vi "Validate DAQ model.vi"(8 "error in (no error)":errorcluster, 10 "Desired model":string[](array[string]), 11 "DAQ Module ID":i32) -> (0 "error out":errorcluster, 2 "Device found":string, 3 "Is model valid?":bool)   [LabVIEW 2020]
doc: "Validates whether the DAQ connected at the port is a desired DAQ model."
uses:
  NI_DAQ/Libraries/NI DAQ/NI DAQ.lvlib
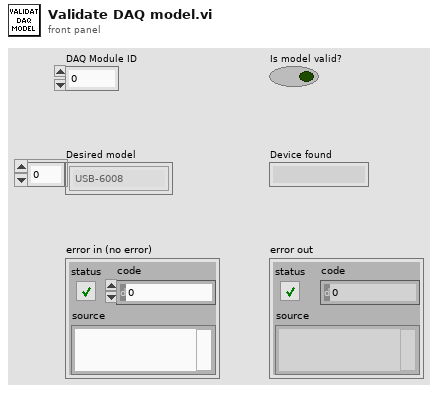
[diagram p1: front panel]
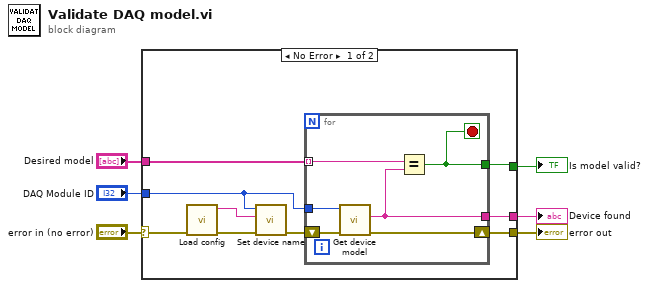
[diagram p0: block diagram]
diagram:
  n1 = case shown="No Error" "error in (no error)" {
    selector: "error in (no error)" -> [w10 w22]
    tunnel: [w7 _] -> w6
    tunnel: "DAQ Module ID" -> [w15 _]
    tunnel: [w14 w22] -> w4
    tunnel: "Desired model" -> [w8 _]
    tunnel: [w9 _] -> w1
    frame No Error {
      n2 = call "Load config.vi"("error in (no error)"=w10) -> ("error out"=w11:errorcluster, "DAQ Port"=w12:tag)  [unwired: 9 in]
      n3 = call "Set device name.vi"("error in"=w11, "Device name"=w12, "Module ID"=w15) -> ("error out"=w13:errorcluster)  [unwired: 8 in]
      n4 = for {
        tunnel: w15 -> [w21]
        tunnel: [w17] -> w9
        shift-right: [w20] -> w14
        shift-left: w13 -> [w19]
        tunnel: w8 -> [w18] mode=indexing
        tunnel: [w16] -> w7
        stop <- w16 stop-if-true
        n5 = call "Get device model.vi"("error in"=w19, "Module ID"=w21) -> ("error out"=w20:errorcluster, "Device model"=w17:string)  [unwired: 7 in, 1 out]
        n6 = Equal?(x=w18, y=w17) -> (x = y?=w16:bool)
      }
    }
    frame Error {
    }
  }
  "Is model valid?" <- w6
  "error out" <- w4
  "Device found" <- w1
